vi "Write Pulse Initial.vi"(8 "error in":errorcluster, 10 "Pulse Initial":dbl, 11 "3300 in":refnum<class "3300.lvclass">) -> (0 "error out":errorcluster, 3 "3300 out":refnum<class "3300.lvclass">)   [LabVIEW 2019, in "3300.lvlib" / "3300.lvclass"]
uses:
  Library/3300.lvclass
  C:/Users/Public/Documents/Development/builds/Instruments/Electronic Load.lvlibp/Library/Electronic Load.lvclass
  builds/Instruments/Electronic Load.lvlibp/Accessors/Trigger/Read Pulse Mode.vi
  builds/Instruments/Electronic Load.lvlibp/Library/Electronic Load.lvclass
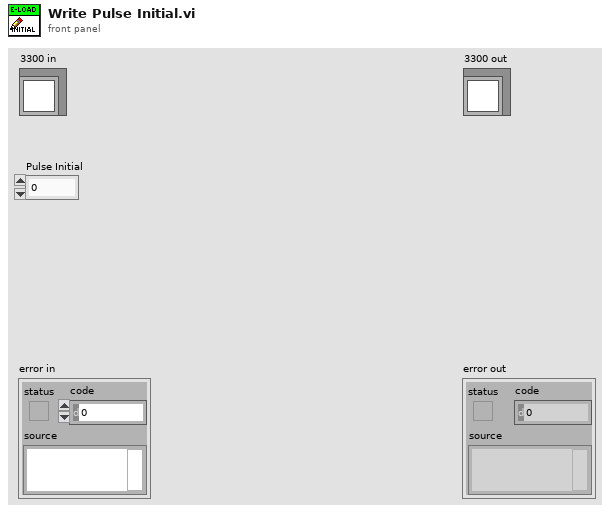
[diagram p1: front panel]
types:
  T1 = typedef "Electronic Load.lvlibp/Electronic Load.lvclass/E-Load Mode.ctl" = enum16{"Current", "Resistance", "Voltage"}
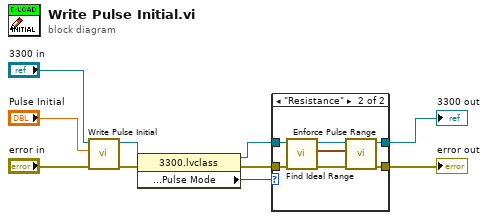
[diagram p0: block diagram]
diagram:
  n1 = call-parent "Write Pulse Initial.vi"("error in"="error in", "Pulse Initial"="Pulse Initial", "Electronic Load in"="3300 in") -> ("error out"=w4:errorcluster, "Electronic Load out"=w5:refnum<class "3300.lvclass">)  [unwired: 7 in]
  n2 = property class="3300.lvclass"(reference=w5, error in=w4) -> (reference out=w2:refnum<class "3300.lvclass">, error out=w3:errorcluster, "Accessors:Settings:Pulse:Pulse Mode"=w1:T1)
  n3 = case shown="\"Resistance\"" w1 {
    tunnel: [w11 w16] -> w7
    tunnel: [w12 w15] -> w6
    tunnel: w3 -> [w11 w14]
    tunnel: w2 -> [w12 w13]
    frame "Current", Default {
    }
    frame "Resistance" {
      n4 = call "Find Ideal Range.vi"("error in"=w14, "3300 in"=w13) -> ("error out"=w19:errorcluster, "Ideal Range"=w18:cluster{"Low":dbl, "High":dbl}, "3300 out"=w17:refnum<class "3300.lvclass">)  [unwired: 7 in]
      n5 = call "Enforce Pulse Range.vi"("error in"=w19, "Ideal Range"=w18, "3300 in"=w17) -> ("error out"=w16:errorcluster, "3300 out"=w15:refnum<class "3300.lvclass">)  [unwired: 7 in]
    }
  }
  "error out" <- w7
  "3300 out" <- w6
